vi "Soft Start.vi"(0 "Joysticks":T2, 1 "Slew Rates":T1={"X-Slew"=0.1, "Y-Slew Go"=0.1, "Z-Slew"=0.1}) -> (2 "X-axis drive":dbl, 3 "Y-axis drive":dbl, 4 "Z-axis drive":dbl)   [LabVIEW 2016]
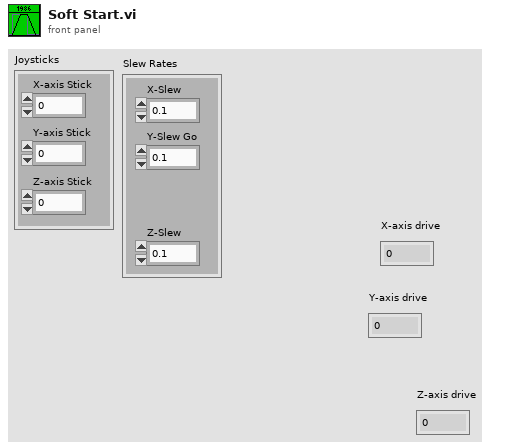
[diagram p1: front panel]
types:
  T1 = cluster{"X-Slew":dbl, "Y-Slew Go":dbl, "Z-Slew":dbl}
  T2 = cluster{"X-axis Stick":dbl, "Y-axis Stick":dbl, "Z-axis Stick":dbl}
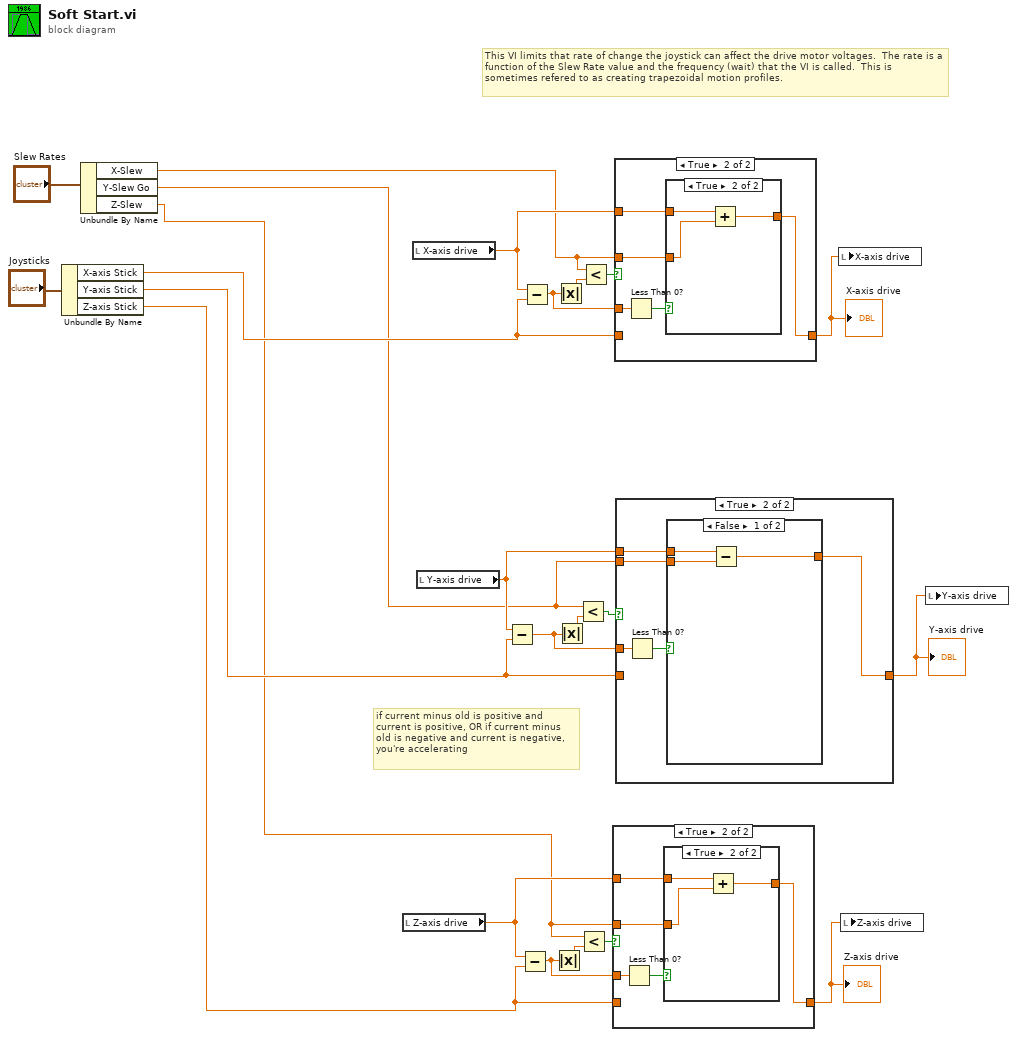
[diagram p0: block diagram]
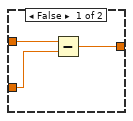
[diagram p3: hidden frame]
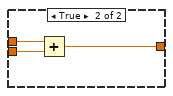
[diagram p5: hidden frame]
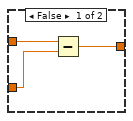
[diagram p7: hidden frame]
diagram:
  # "if current minus old is positive and\ncurrent is positive, OR if current minus\nold is negative and current is negative,\nyou're accelerating"
  # "This VI limits that rate of change the joystick can affect the drive motor voltages.  The rate is a function of the Slew Rate value and the frequency (wait) that the VI is called.  This is sometimes refered to as creating trapezoidal motion profiles."
  n1 = Unbundle By Name("Joysticks") -> ("X-axis Stick"=w8:dbl, "Y-axis Stick"=w4:dbl, "Z-axis Stick"=w7:dbl)
  n2 = Unbundle By Name("Slew Rates") -> ("X-Slew"=w5:dbl, "Y-Slew Go"=w1:dbl, "Z-Slew"=w2:dbl)
  n3 = local read "Z-axis drive"() -> (w10:dbl)
  n4 = local read "X-axis drive"() -> (w19:dbl)
  n5 = local read "Y-axis drive"() -> (w15:dbl)
  n6 = Subtract(x=w15, y=w4) -> (x-y=w3:dbl)
  n7 = Subtract(x=w10, y=w7) -> (x-y=w12:dbl)
  n8 = Subtract(x=w19, y=w8) -> (x-y=w21:dbl)
  n9 = Absolute Value(x=w12) -> (abs(x)=w14:dbl)
  n10 = Absolute Value(x=w21) -> (abs(x)=w23:dbl)
  n11 = Absolute Value(x=w3) -> (abs(x)=w18:dbl)
  n12 = Less?(x=w1, y=w18) -> (x < y?=w17:bool)
  n13 = Less?(x=w2, y=w14) -> (x < y?=w13:bool)
  n14 = Less?(x=w5, y=w23) -> (x < y?=w22:bool)
  n15 = case shown="True" w13 {
    tunnel: [w24 w25] -> w11
    tunnel: w7 -> [w24 _]
    tunnel: w12 -> [_ w29]
    tunnel: w10 -> [_ w27]
    tunnel: w2 -> [_ w26]
    frame False {
    }
    frame True {
      n16 = Less Than 0?(x=w29) -> (x < 0?=w28:bool)
      n17 = case shown="True" w28 {
        tunnel: w27 -> [w32 w35]
        tunnel: w26 -> [w30 w33]
        tunnel: [w31 w34] -> w25
        frame False {
          n18 = Subtract(x=w32, y=w30) -> (x-y=w31:dbl)
        }
        frame True {
          n19 = Add(x=w35, y=w33) -> (x+y=w34:dbl)
        }
      }
    }
  }
  "Z-axis drive" <- w11
  n20 = case shown="True" w22 {
    tunnel: [w36 w37] -> w20
    tunnel: w8 -> [w36 _]
    tunnel: w21 -> [_ w41]
    tunnel: w19 -> [_ w39]
    tunnel: w5 -> [_ w38]
    frame False {
    }
    frame True {
      n21 = Less Than 0?(x=w41) -> (x < 0?=w40:bool)
      n22 = case shown="True" w40 {
        tunnel: w39 -> [w44 w47]
        tunnel: w38 -> [w42 w45]
        tunnel: [w43 w46] -> w37
        frame False {
          n23 = Subtract(x=w44, y=w42) -> (x-y=w43:dbl)
        }
        frame True {
          n24 = Add(x=w47, y=w45) -> (x+y=w46:dbl)
        }
      }
    }
  }
  "X-axis drive" <- w20
  n25 = case shown="True" w17 {
    tunnel: [w48 w50] -> w16
    tunnel: w4 -> [w48 _]
    tunnel: w3 -> [_ w53]
    tunnel: w15 -> [_ w51]
    tunnel: w1 -> [_ w49]
    frame False {
    }
    frame True {
      n26 = Less Than 0?(x=w53) -> (x < 0?=w52:bool)
      n27 = case shown="False" w52 {
        tunnel: w51 -> [w56 w59]
        tunnel: [w55 w58] -> w50
        tunnel: w49 -> [w54 w57]
        frame False {
          n28 = Subtract(x=w56, y=w54) -> (x-y=w55:dbl)
        }
        frame True {
          n29 = Add(x=w59, y=w57) -> (x+y=w58:dbl)
        }
      }
    }
  }
  "Y-axis drive" <- w16
  n30 = local write "X-axis drive"(w20) -> ()
  n31 = local write "Z-axis drive"(w11) -> ()
  n32 = local write "Y-axis drive"(w16) -> ()
